vi "Write Sequence State Msg.vi"(8 "error in (no error)":errorcluster, 10 "HIJ Vision Camera App.lvlib:Sequence State Msg.lvclass":refnum<class "Sequence State Msg.lvclass">, 11 "HIJ Vision Camera App in":refnum<class "HIJ Vision Camera App.lvclass">) -> (0 "error out":errorcluster, 3 "HIJ Vision Camera App out":refnum<class "HIJ Vision Camera App.lvclass">)   [LabVIEW 2014, in "HIJ Vision Camera App.lvlib" / "HIJ Vision Camera App.lvclass"]
uses:
  HIJ Vision Camera App.lvclass
  HIJ Vision Camera App Messages/Sequence State Msg/Sequence State Msg.lvclass
  HIJ Vision Camera App.lvclass/HIJ Vision Camera App.ctl
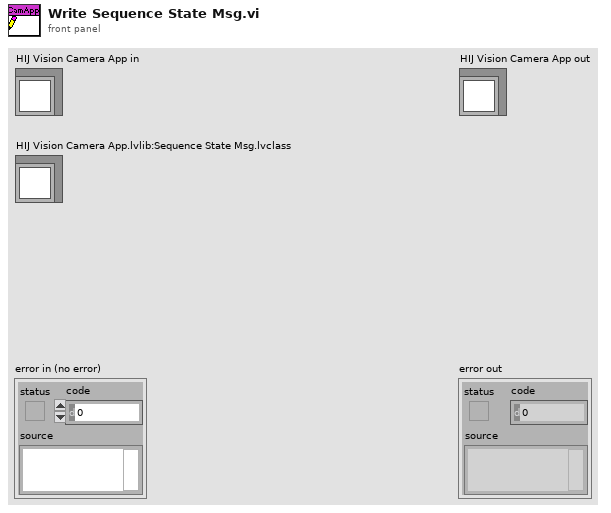
[diagram p1: front panel]
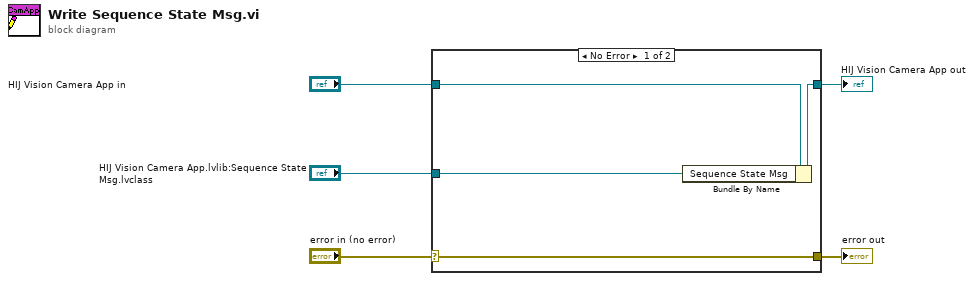
[diagram p0: block diagram]
diagram:
  n1 = case shown="No Error" "error in (no error)" {
    selector: "error in (no error)" -> [w9 w10]
    tunnel: [w9 w10] -> w4
    tunnel: [w7 w11] -> w2
    tunnel: "HIJ Vision Camera App in" -> [w8 w11]
    tunnel: "HIJ Vision Camera App.lvlib:Sequence State Msg.lvclass" -> [w6 _]
    frame No Error {
      n2 = Bundle By Name(cluster=w8, "Sequence State Msg"=w6) -> (w7:refnum<class "HIJ Vision Camera App.lvclass">)
    }
    frame Error {
    }
  }
  "error out" <- w4
  "HIJ Vision Camera App out" <- w2
